vi "Move single motor.vi"(8 "error in (no error)":errorcluster, 10 "Motor params":T1, 11 "DAQ Module ID":i32) -> (0 "error out":errorcluster)   [LabVIEW 2020]
uses:
  Motor direction ---typedef.ctl
  NI_DAQ/Libraries/NI DAQ/NI DAQ.lvlib
  NI_DAQ/Libraries/NI DAQ/Controls/Motor controls---typedef.ctl
  Motor params ---typedef.ctl
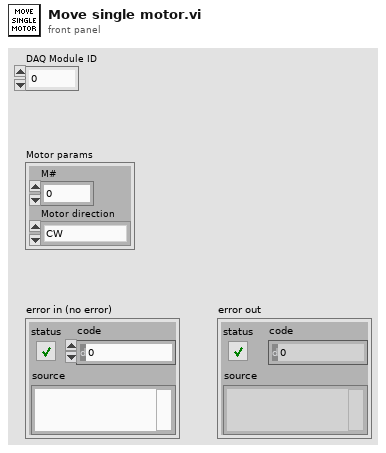
[diagram p1: front panel]
types:
  T1 = typedef "Motor params ---typedef.ctl" = cluster{"M#":i32, "Motor direction":T2}
  T2 = typedef "Motor direction ---typedef.ctl" = enum16{"CW", "CCW"}
  T3 = typedef "Motor controls---typedef.ctl" = cluster{"EN1":bool, "DIR1":bool, "EN2":bool, "DIR2":bool, "TOG":bool}
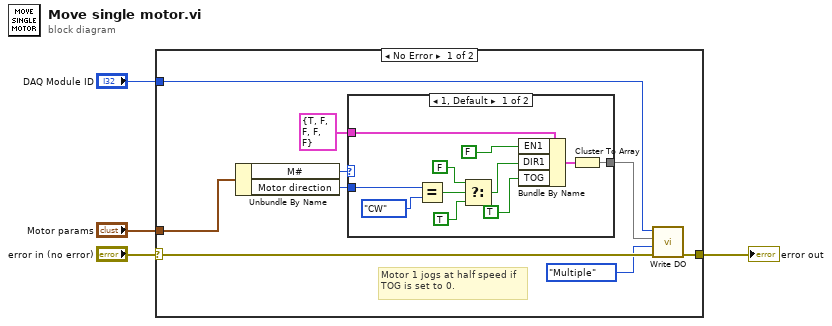
[diagram p0: block diagram]
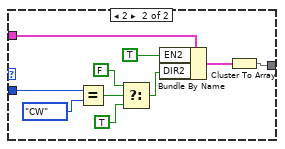
[diagram p2: hidden frame]
diagram:
  n1 = case shown="No Error" "error in (no error)" {
    selector: "error in (no error)" -> [w10 w35]
    tunnel: [w11 w35] -> w4
    tunnel: "DAQ Module ID" -> [w9 _]
    tunnel: "Motor params" -> [w7 _]
    frame No Error {
      # "Motor 1 jogs at half speed if TOG is set to 0."
      n2 = Unbundle By Name(w7) -> ("M#"=w8:i32, "Motor direction"=w13:T2)
      n3 = case shown="1, Default" w8 {
        tunnel: T3 {"EN1"=TRUE, "DIR1"=FALSE, "EN2"=FALSE, "DIR2"=FALSE, "TOG"=FALSE} ("Motor control") -> [w24 w34]
        tunnel: w13 -> [w22 w32]
        tunnel: [w15 w25] -> w6
        frame 1, Default {
          n4 = Equal?(x=w22, y=Motor_direction_---typedef."CW") -> (x = y?=w20:bool)
          n5 = Select(t=FALSE ("EN1"), s=w20, f=TRUE) -> (s? t:f=w17:bool)
          n6 = Bundle By Name(cluster=w24, "EN1"=FALSE, "DIR1"=w17, "TOG"=TRUE) -> (w16:T3)
          n7 = Cluster To Array(cluster=w16) -> (array=w15:bool[])
        }
        frame 2 {
          n8 = Equal?(x=w32, y=Motor_direction_---typedef."CW") -> (x = y?=w30:bool)
          n9 = Select(t=FALSE ("EN1"), s=w30, f=TRUE) -> (s? t:f=w27:bool)
          n10 = Bundle By Name(cluster=w34, "EN2"=TRUE ("EN1"), "DIR2"=w27) -> (w26:T3)
          n11 = Cluster To Array(cluster=w26) -> (array=w25:bool[])
        }
      }
      n12 = call "Write DO.vi"("error in"=w10, "Samples"=enum16{"Single", "Multiple"}."Multiple", "Data"=w6, "Module ID"=w9) -> ("error out"=w11:errorcluster)  [unwired: 7 in]
    }
    frame Error {
    }
  }
  "error out" <- w4
